vi "Main.vi"(11 "Module Admin":refnum<class "Delacor_lib_QMH_Module Admin.lvclass">) -> ()   [LabVIEW 2018, in "MB switches Module.lvlib"]
doc: "This template is based off of the Queued Message Handler design pattern and the Queued Message Handler project template that ships with LabVIEW.\n\nThe main difference is that the queue is private to this module and communication between modules is performed via Broadcast and Request events.\n\nRequest events are wrapped in public API methods and are handled in the Event Handling Loop (EHL) of this VI. Any module can register for Broadcast events sent by this module. The EHL generates messages based on user interface actions.\n\nThe Message Handling Loop (MHL) processes messages generated by the EHL, or by other messages. The messages are string values, so new messages can be added easily to the Message Cases case structure in the MHL. Each message cluster can also provide an optional value for Message Data, which is a variant that can be converted to whatever message-specific data is required.\n_____\nBased on DQMH Project Template 6.0.0.91."
uses:
  MB switches Module.lvlib
  <vilib>/Delacor/Delacor QMH/Libraries/Module Admin_class/Delacor_lib_QMH_Module Admin.lvclass
  Module Data--cluster.ctl
  <vilib>/NI/Modbus Library/API/Master/Modbus Master.lvclass
  Do Something Else and Wait for Reply Argument--cluster.ctl
  Do Something Else and Wait (Reply Payload)--cluster.ctl
  <vilib>/Delacor/Delacor QMH/Libraries/Message Queue_class/Delacor_lib_QMH_Message Queue.lvclass/Delacor_lib_QMH_Message Queue.ctl
  Stop Argument--cluster.ctl
  <vilib>/Delacor/Delacor QMH/Libraries/Module Admin_class/Delacor_lib_QMH_Module Admin.lvclass/Delacor_lib_QMH_Module Admin.ctl
  inst.Counter Argument--cluster.ctl
  inst.Counter (Reply Payload)--cluster.ctl
  inst.Optos Argument--cluster.ctl
  inst.Optos (Reply Payload)--cluster.ctl
  inst.mux10_1 Argument--cluster.ctl
  inst.mux6_1(3wires) Argument--cluster.ctl
  inst.Open Argument--cluster.ctl
  inst.Close Argument--cluster.ctl
  DMM I 0.5_10 Argument--cluster.ctl
  <vilib>/Utility/miscctls.llb/LVPointTypeDef.ctl
  Instrument Drivers/LV_driver_MBrelay/type defs/FGV enum.ctl
  <vilib>/Delacor/Delacor QMH/Libraries/Message Queue_class/Delacor_lib_QMH_Enqueue Message (Single).vi
  <vilib>/Delacor/Delacor QMH/Libraries/Module Admin_class/Delacor_lib_QMH_Get External Launch.vi
  <vilib>/Utility/error.llb/Error Cluster From Error Code.vi
  <vilib>/ErrorRing/Error Ring.xnode
  <vilib>/Delacor/Delacor QMH/Libraries/Message Queue_class/Delacor_lib_QMH_Message Queue.lvclass
  Instrument Drivers/LV_driver_MBrelay/MB Relay.lvlib
panel:
  in  "VISA resource name":refnum<visa-resource-name>="COM4"
  out "error out":errorcluster
  out "Status":string
  in  "Simulate MHL Error":bool
  in  "Simulate EHL Error":bool
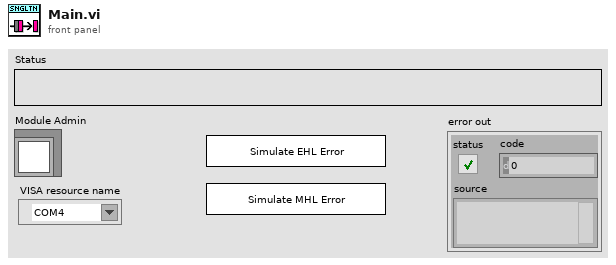
[diagram p1: front panel]
types:
  T1 = typedef "MB switches Module.lvlib/Request Events--cluster.ctl" = cluster{"Stop Module":refnum<user-event>, "Do Something Else and Wait for Reply":refnum<user-event>, "Show Panel":refnum<user-event>, "Hide Panel":refnum<user-event>, "Get Module Execution Status":refnum<user-event>, "Show Diagram":refnum<user-event>, "inst.Counter":refnum<user-event>, "inst.Open":refnum<user-event>, "inst.Close":refnum<user-event>, "inst.Optos":refnum<user-event>, "inst.mux10_1":refnum<user-event>, "inst.mux6_1(3wires)":refnum<user-event>, "DMM I 0.5_10":refnum<user-event>}
  T2 = typedef "MB switches Module.lvlib/Module Data--cluster.ctl" = cluster{"Status":string, "Modbus Master ref":refnum<class "Modbus Master.lvclass">}
  T3 = typedef "MB switches Module.lvlib/Do Something Else and Wait for Reply Argument--cluster.ctl" = cluster{"Do Something Else Msg":string, "X":dbl, "Wait Notifier":refnum<notifier>, "wait for reply":bool}
  T4 = enum32{"invalid lock state", "Not Locked", "Locked (No Password)", "Password-protected"}
  T5 = typedef "MB switches Module.lvlib/Stop Argument--cluster.ctl" = cluster{"Origin":string, "Exit via Stop Module Req?":bool, "Wait for Module to stop?":bool}
  T6 = typedef "MB switches Module.lvlib/inst.Counter Argument--cluster.ctl" = cluster{"Wait Notifier":refnum<notifier>, "wait for reply":bool}
  T7 = typedef "MB switches Module.lvlib/inst.Optos Argument--cluster.ctl" = cluster{"Wait Notifier":refnum<notifier>, "wait for reply":bool}
  T8 = typedef "MB switches Module.lvlib/inst.mux10_1 Argument--cluster.ctl" = cluster{"mux10_1(x6)_encode":enum16{"mux10_1_channel0", "mux10_1_channel1", "mux10_1_channel2", "mux10_1_channel3", "mux10_1_channel4", "mux10_1_channel5", "mux10_1_channel6", "mux10_1_channel7", "mux10_1_channel8", "mux10_1_channel9", "mux10_1_channel10"}}
  T9 = typedef "MB switches Module.lvlib/inst.mux6_1(3wires) Argument--cluster.ctl" = cluster{"mux6_1(3wires)_encode":enum16{"mux6-1_channel0", "mux6_1_channel1_0", "mux6_1_channel1_1", "mux6-1_channel1_2", "mux6_1_channel1_3", "mux6_1_channel2_0", "mux6_1_channel2_1", "mux6_1_channel2_2", "mux6_1_channel2_3", "mux6_1_channel3_0", "mux6_1_channel3_1", "mux6_1_channel3_2", "mux6_1_channel3_3", "mux6_1_channel4_0", "mux6_1_channel4_1", "mux6_1_channel4_2", "mux6_1_channel4_3", "mux6_1_channel5_0", "mux6_1_channel5_1", "mux6_1_channel5_2", "mux6_1_channel5_3", "mux6_1_channel6_0", "mux6_1_channel6_1", "mux6_1_channel6_2", "mux6_1_channel6_3"}}
  T10 = typedef "MB switches Module.lvlib/DMM I 0.5_10 Argument--cluster.ctl" = cluster{"mux2-1(DMM I) encode":enum16{"DMM I (0.5)", "DMM I (12)"}}
  T11 = typedef "LVPointTypeDef.ctl" = cluster{"Horizontal":i16, "Vertical":i16}
  T12 = enum32{"Invalid", "Standard", "Closed", "Hidden", "Minimized", "Maximized"}
  T13 = typedef "MB switches Module.lvlib/Do Something Else and Wait (Reply Payload)--cluster.ctl" = cluster{"Value":dbl, "error":errorcluster}
  T14 = typedef "MB switches Module.lvlib/inst.Counter (Reply Payload)--cluster.ctl" = cluster{"counter":u16, "inst.Counter_error":errorcluster}
  T15 = typedef "MB switches Module.lvlib/inst.Open Argument--cluster.ctl" = cluster{"VISA resource name":refnum<visa-resource-name>}
  T16 = typedef "MB Relay.lvlib/FGV enum.ctl" = enum16{"Write", "Read", "All OFF", "All ON"}
  T17 = typedef "MB switches Module.lvlib/inst.Close Argument--cluster.ctl" = cluster{"Boolean":bool}
  T18 = typedef "MB switches Module.lvlib/inst.Optos (Reply Payload)--cluster.ctl" = cluster{"Optos":bool[], "inst.Optos_error":errorcluster}
  T19 = enum16{"mux10_1_channel0", "mux10_1_channel1", "mux10_1_channel2", "mux10_1_channel3", "mux10_1_channel4", "mux10_1_channel5", "mux10_1_channel6", "mux10_1_channel7", "mux10_1_channel8", "mux10_1_channel9", "mux10_1_channel10"}
  T20 = enum16{"mux6-1_channel0", "mux6_1_channel1_0", "mux6_1_channel1_1", "mux6-1_channel1_2", "mux6_1_channel1_3", "mux6_1_channel2_0", "mux6_1_channel2_1", "mux6_1_channel2_2", "mux6_1_channel2_3", "mux6_1_channel3_0", "mux6_1_channel3_1", "mux6_1_channel3_2", "mux6_1_channel3_3", "mux6_1_channel4_0", "mux6_1_channel4_1", "mux6_1_channel4_2", "mux6_1_channel4_3", "mux6_1_channel5_0", "mux6_1_channel5_1", "mux6_1_channel5_2", "mux6_1_channel5_3", "mux6_1_channel6_0", "mux6_1_channel6_1", "mux6_1_channel6_2", "mux6_1_channel6_3"}
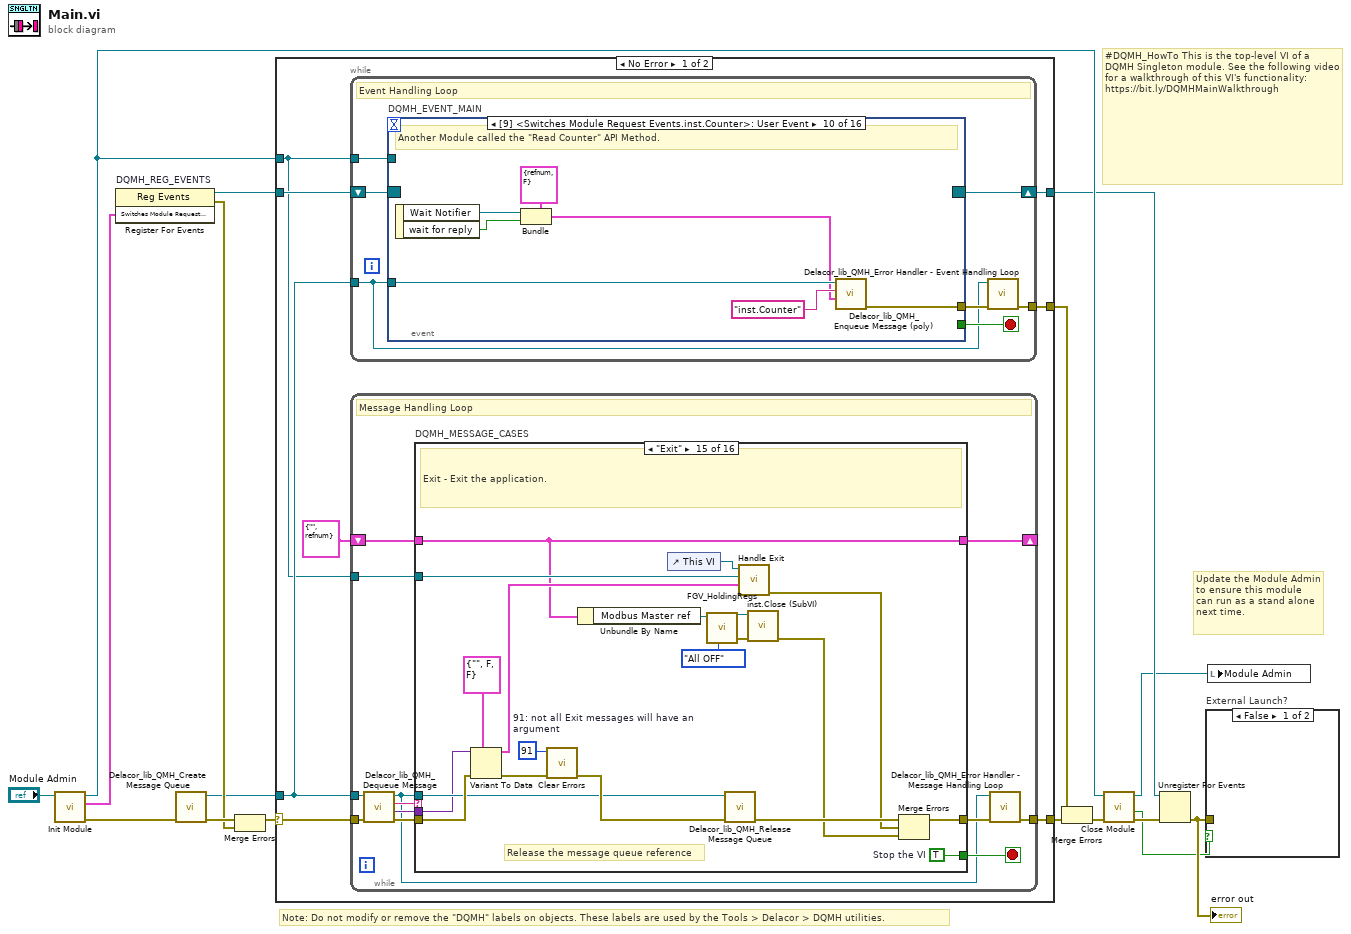
[diagram p0: block diagram]
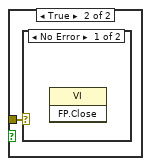
[diagram p2: hidden frame]
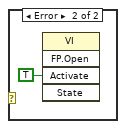
[diagram p3: hidden frame]
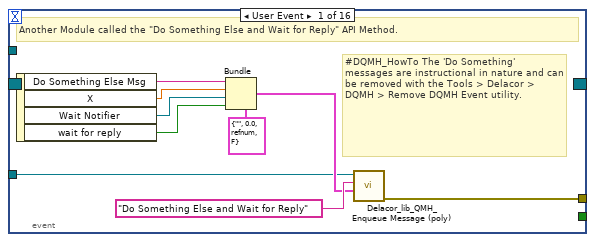
[diagram p4: hidden frame]
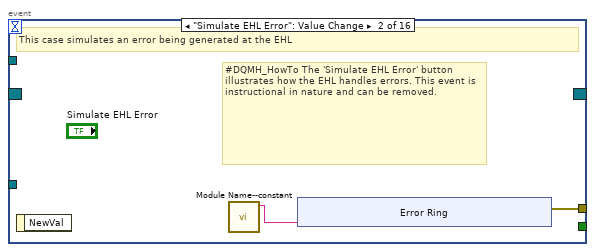
[diagram p5: hidden frame]
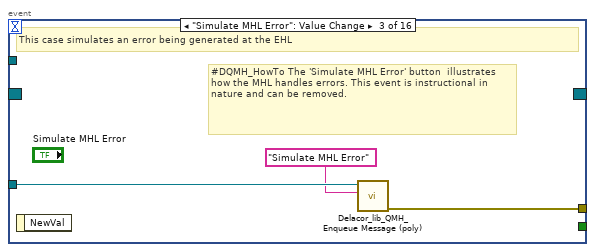
[diagram p6: hidden frame]
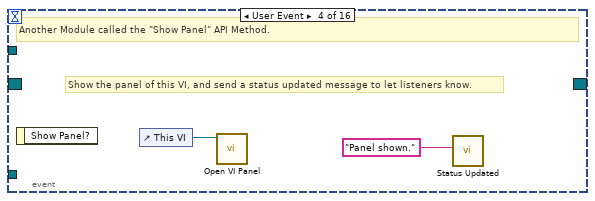
[diagram p7: hidden frame]
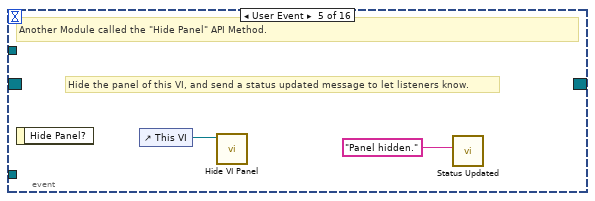
[diagram p8: hidden frame]
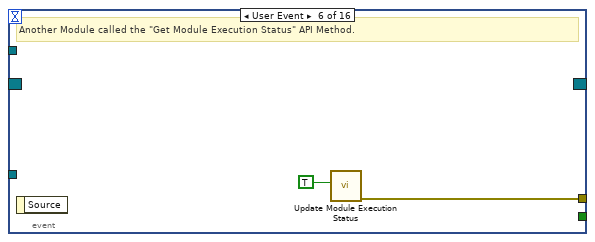
[diagram p9: hidden frame]
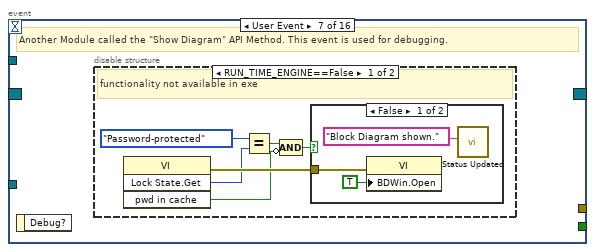
[diagram p10: hidden frame]
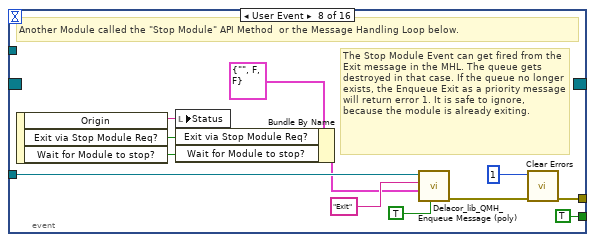
[diagram p13: hidden frame]
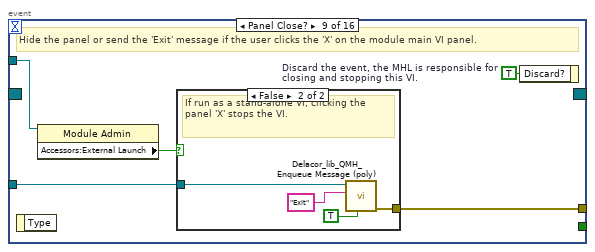
[diagram p14: hidden frame]
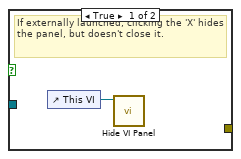
[diagram p15: hidden frame]
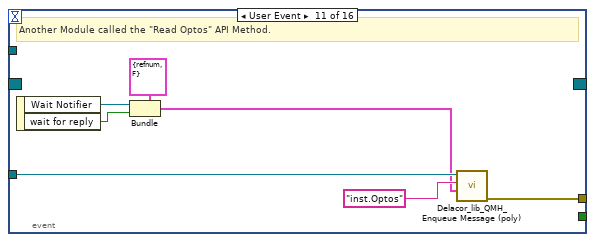
[diagram p16: hidden frame]
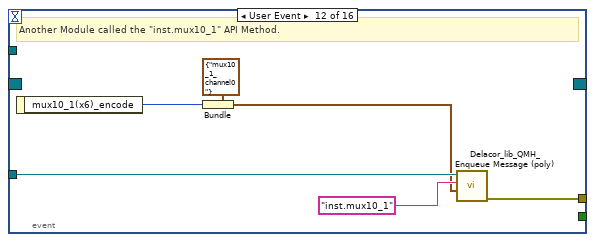
[diagram p17: hidden frame]
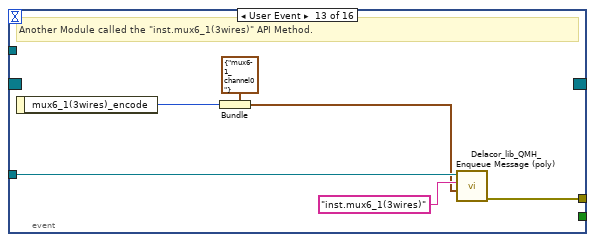
[diagram p18: hidden frame]
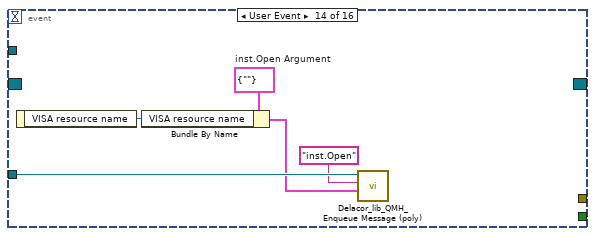
[diagram p19: hidden frame]
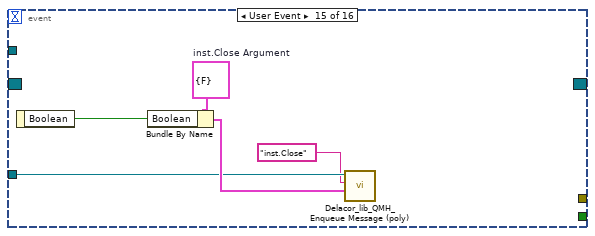
[diagram p20: hidden frame]
diagram:
  # "#DQMH_HowTo This is the top-level VI of a DQMH Singleton module. See the following video for a walkthrough of this VI's functionality: https://bit.ly/DQMHMainWalkthrough"
  # "Note: Do not modify or remove the \"DQMH\" labels on objects. These labels are used by the Tools > Delacor > DQMH utilities."
  # "Update the Module Admin to ensure this module can run as a stand alone next time."
  n1 = call "Init Module.vi"("Singleton Module Admin in"="Module Admin") -> ("error out"=w16:errorcluster, "Switches Module Request Events"=w2:T1, "Singleton Module Admin out"=w8:refnum<class "Delacor_lib_QMH_Module Admin.lvclass">)  [unwired: 8 in]
  n2 = register-events "DQMH_REG_EVENTS"(w2) -> (reference out=w1:refnum<event-registration>, error out=w9:errorcluster)  [unwired: 2 in]
  n3 = call <vilib>:"Delacor_lib_QMH_Create Message Queue.vi"("error in"=w16) -> ("error out"=w11:errorcluster, "Message Queue"=w6:refnum<class "Delacor_lib_QMH_Message Queue.lvclass">)  [unwired: 9 in]
  n4 = Merge Errors(w11, w9) -> (w10:errorcluster)
  n5 = case shown="No Error" w10 {
    selector: w10 -> [w23 w357]
    tunnel: [w25 w356] -> w17
    tunnel: [w22 w362] -> w7
    tunnel: w1 -> [w20 w362]
    tunnel: w6 -> [w19 w355]
    tunnel: [w24 _] -> w14
    tunnel: w8 -> [w18 w358]
    frame No Error {
      n6 = while {
        tunnel: w19 -> [w26]
        shift-right: [w29] -> w22
        shift-left: w20 -> [w30]
        tunnel: [w31] -> w24
        tunnel: w18 -> [w27]
        stop <- w28 stop-if-true
        # "Event Handling Loop"
        n7 = event "DQMH_EVENT_MAIN" shown="[9] <Switches Module Request Events.inst.Counter>: User Event" {
          selector: w30 -> [_ _ _ _ _ _ _ _ _ _ _ _ _ _ _ _]
          dyn-events: [_ _ _ _ _ _ _ _ _ _ _ _ _ _ _ _] -> w29
          timeout: _ -> [_ _ _ _ _ _ _ _ _ _ _ _ _ _ _ _]
          tunnel: [_ _ _ _ _ _ _ TRUE ("Discard?") _ _ _ _ _ _ _ _] -> w28
          tunnel: w26 -> [w34 _ w52 _ _ _ _ w76 w83 w97 w104 w110 w116 w121 w123 w132]
          tunnel: [w41 w43 w53 _ _ w59 _ w79 w85 w91 w98 w105 w111 _ _ w127] -> w32
          tunnel: w27 -> [_ _ _ _ _ _ _ _ w82 _ _ _ _ _ _ _]
          event User Event {
            # "#DQMH_HowTo The 'Do Something' messages are instructional in nature and can be removed with the Tools > Delacor > DQMH > Remove DQMH Event utility."
            # "Another Module called the \"Do Something Else and Wait for Reply\" API Method."
            n8 = event-data() -> ("Do Something Else Msg"=w37:string, "X"=w36:dbl, "Wait Notifier"=w35:refnum<notifier>, "wait for reply"=w33:bool)  [unwired: 1 in]
            n9 = Bundle(cluster=T3 {"Do Something Else Msg"="", "X"=0.0, "Wait Notifier"=refnum, "wait for reply"=FALSE} ("Do Something Else and Wait for Reply Argument"), "Do Something Else Msg"=w37, "X"=w36, "Wait Notifier"=w35, "wait for reply"=w33) -> (w38:T3)
            n10 = call-poly <vilib>:"Delacor_lib_QMH_Enqueue Message (poly).vi"("Message Data"=w38, "Message"="Do Something Else and Wait for Reply", "Message Queue in"=w34) -> ("error out"=w41:errorcluster)  [unwired: 7 in, 1 out]
          }
          event "Simulate EHL Error": Value Change {
            # "#DQMH_HowTo The 'Simulate EHL Error' button  illustrates how the EHL handles errors. This event is instructional in nature and can be removed."
            # "This case simulates an error being generated at the EHL"
            n11 = event-data() -> ()  [unwired: 1 in, 1 out]
            n12 = call "Module Name--constant.vi"() -> ("Module Name"=w42:string)  [unwired: 11 in]
            n13 = xnode "Error Ring"("parameter 0"=w42) -> ("error out"=w43:errorcluster)
          }
          event "Simulate MHL Error": Value Change {
            # "#DQMH_HowTo The 'Simulate MHL Error' button  illustrates how the MHL handles errors. This event is instructional in nature and can be removed."
            # "This case simulates an error being generated at the EHL"
            n14 = event-data() -> ()  [unwired: 1 in, 1 out]
            n15 = call-poly <vilib>:"Delacor_lib_QMH_Enqueue Message (poly).vi"("Message"="Simulate MHL Error", "Message Queue in"=w52) -> ("error out"=w53:errorcluster)  [unwired: 8 in, 1 out]
          }
          event User Event {
            # "Show the panel of this VI, and send a status updated message to let listeners know."
            # "Another Module called the \"Show Panel\" API Method."
            n16 = event-data() -> ()  [unwired: 1 in, 1 out]
            n17 = control-ref of="This VI"() -> (w55:refnum<vi>)
            n18 = call "Open VI Panel.vi"("VI"=w55) -> ()  [unwired: 10 in, 1 out]
            n19 = call "Status Updated.vi"("Status"="Panel shown." ("format string")) -> ()  [unwired: 10 in, 1 out]
          }
          event User Event {
            # "Hide the panel of this VI, and send a status updated message to let listeners know."
            # "Another Module called the \"Hide Panel\" API Method."
            n20 = event-data() -> ()  [unwired: 1 in, 1 out]
            n21 = control-ref of="This VI"() -> (w57:refnum<vi>)
            n22 = call "Hide VI Panel.vi"("VI"=w57) -> ()  [unwired: 10 in, 1 out]
            n23 = call "Status Updated.vi"("Status"="Panel hidden." ("format string")) -> ()  [unwired: 10 in, 1 out]
          }
          event User Event {
            # "Another Module called the \"Get Module Execution Status\" API Method."
            n24 = event-data() -> ()  [unwired: 1 in, 1 out]
            n25 = call "Update Module Execution Status.vi"("Running?"=TRUE) -> ("error out"=w59:errorcluster)  [unwired: 10 in]
          }
          event User Event {
            # "Another Module called the \"Show Diagram\" API Method. This event is used for debugging."
            n26 = event-data() -> ()  [unwired: 1 in, 1 out]
            n27 = disable-structure shown="RUN_TIME_ENGINE==False" {
              frame condition #0 (active) {
                # "functionality not available in exe"
                n28 = invoke class="VI" method="Lock State.Get"() -> (error out=w65:errorcluster, "Get Lock State"=w64:T4, "pwd in cache"=w61:bool)  [unwired: 4 in, 1 out]
                n29 = Equal?(x=T4."Password-protected", y=w64) -> (x = y?=w62:bool)
                n30 = Compound Arithmetic op=AND(w62, invert w61) -> (w60:bool)
                n31 = case shown="False" w60 {
                  tunnel: w65 -> [w68 _]
                  frame False {
                    n32 = property class="VI"(error in=w68, "BDWin.Open"=TRUE ("Block Diagram Window:Open")) -> ()  [unwired: 1 in, 2 out]
                    n33 = call "Status Updated.vi"("Status"="Block Diagram shown." ("format string")) -> ()  [unwired: 10 in, 1 out]
                  }
                  frame True {
                    # "Password-protected VI, and the password is not in the cache. Do not show the diagram."
                  }
                }
              }
              frame condition #1 {
              }
            }
          }
          event User Event {
            # "The Stop Module Event can get fired from the Exit message in the MHL. The queue gets destroyed in that case. If the queue no longer exists, the Enqueue Exit as a priority message will return error 1. It is safe to ignore, because the module is already exiting."
            # "Another Module called the \"Stop Module\" API Method  or the Message Handling Loop below."
            n34 = event-data() -> ("Origin"=w75:string, "Exit via Stop Module Req?"=w71:bool, "Wait for Module to stop?"=w70:bool)  [unwired: 1 in]
            n35 = local write "Status"(w75) -> ()
            n36 = Bundle By Name(cluster=T5 {"Origin"="", "Exit via Stop Module Req?"=FALSE, "Wait for Module to stop?"=FALSE} ("Stop Argument"), "Exit via Stop Module Req?"=w71, "Wait for Module to stop?"=w70) -> (w69:T5)
            n37 = call-poly <vilib>:"Delacor_lib_QMH_Enqueue Message (poly).vi"("Priority Message? (F)"=TRUE, "Message Data"=w69, "Message"="Exit", "Message Queue in"=w76) -> ("error out"=w80:errorcluster)  [unwired: 6 in, 1 out]
            n38 = call <vilib>:"Clear Errors.vi"("error in (no error)"=w80, "specific error code to clear (0: all)"=1) -> ("error out"=w79:errorcluster)  [unwired: 4 in, 1 out]
          }
          event Panel Close? {
            w84 = TRUE  # Discard the event, the MHL is responsible for closing and stopping this VI.
            # "Hide the panel or send the 'Exit' message if the user clicks the 'X' on the module main VI panel."
            n39 = event-data() -> ()  [unwired: 1 in, 1 out]
            n40 = property class="Module Admin"(reference=w82) -> ("Accessors:External Launch"=w81:bool)  [unwired: 1 in, 2 out]
            n41 = case shown="False" w81 {
              tunnel: w83 -> [_ w89]
              tunnel: [_ w90] -> w85
              frame True {
                # "If externally launched, clicking the 'X' hides the panel, but doesn't close it."
                n42 = control-ref of="This VI"() -> (w86:refnum<vi>)
                n43 = call "Hide VI Panel.vi"("VI"=w86) -> ()  [unwired: 10 in, 1 out]
              }
              frame False {
                # "If run as a stand-alone VI, clicking the panel 'X' stops the VI."
                n44 = call-poly <vilib>:"Delacor_lib_QMH_Enqueue Message (poly).vi"("Priority Message? (F)"=TRUE, "Message"="Exit", "Message Queue in"=w89) -> ("error out"=w90:errorcluster)  [unwired: 7 in, 1 out]
              }
            }
            n45 = event-data("Discard?"=w84) -> ()  [unwired: 1 in, 1 out]
          }
          event User Event {
            # "Another Module called the \"Read Counter\" API Method."
            n46 = event-data() -> ("Wait Notifier"=w93:refnum<notifier>, "wait for reply"=w92:bool)  [unwired: 1 in]
            n47 = Bundle(cluster=T6 {"Wait Notifier"=refnum, "wait for reply"=FALSE} ("Read Counter Argument"), "Wait Notifier"=w93, "wait for reply"=w92) -> (w94:T6)
            n48 = call-poly <vilib>:"Delacor_lib_QMH_Enqueue Message (poly).vi"("Message Data"=w94, "Message"="inst.Counter", "Message Queue in"=w97) -> ("error out"=w91:errorcluster)  [unwired: 7 in, 1 out]
          }
          event User Event {
            # "Another Module called the \"Read Optos\" API Method."
            n49 = event-data() -> ("Wait Notifier"=w100:refnum<notifier>, "wait for reply"=w99:bool)  [unwired: 1 in]
            n50 = Bundle(cluster=T7 {"Wait Notifier"=refnum, "wait for reply"=FALSE} ("Read Optos Argument"), "Wait Notifier"=w100, "wait for reply"=w99) -> (w101:T7)
            n51 = call-poly <vilib>:"Delacor_lib_QMH_Enqueue Message (poly).vi"("Message Data"=w101, "Message"="inst.Optos", "Message Queue in"=w104) -> ("error out"=w98:errorcluster)  [unwired: 7 in, 1 out]
          }
          event User Event {
            # "Another Module called the \"inst.mux10_1\" API Method."
            n52 = event-data() -> ("mux10_1(x6)_encode"=w106:T19)  [unwired: 1 in]
            n53 = Bundle(cluster=T8 {"mux10_1(x6)_encode"=enum."mux10_1_channel0"} ("inst.mux10_1 Argument"), "mux10_1(x6)_encode"=w106) -> (w107:T8)
            n54 = call-poly <vilib>:"Delacor_lib_QMH_Enqueue Message (poly).vi"("Message Data"=w107, "Message"="inst.mux10_1", "Message Queue in"=w110) -> ("error out"=w105:errorcluster)  [unwired: 7 in, 1 out]
          }
          event User Event {
            # "Another Module called the \"inst.mux6_1(3wires)\" API Method."
            n55 = event-data() -> ("mux6_1(3wires)_encode"=w112:T20)  [unwired: 1 in]
            n56 = Bundle(cluster=T9 {"mux6_1(3wires)_encode"=enum."mux6-1_channel0"} ("inst.mux6_1(3wires) Argument"), "mux6_1(3wires)_encode"=w112) -> (w113:T9)
            n57 = call-poly <vilib>:"Delacor_lib_QMH_Enqueue Message (poly).vi"("Message Data"=w113, "Message"="inst.mux6_1(3wires)", "Message Queue in"=w116) -> ("error out"=w111:errorcluster)  [unwired: 7 in, 1 out]
          }
          event User Event {
            w119 = T15 {"VISA resource name"=""}  # inst.Open Argument
            n58 = event-data() -> ("VISA resource name"=w118:refnum<visa-resource-name>)  [unwired: 1 in]
            n59 = Bundle By Name(cluster=w119, "VISA resource name"=w118) -> (w117:T15)
            n60 = call-poly <vilib>:"Delacor_lib_QMH_Enqueue Message (poly).vi"("Message Data"=w117, "Message"="inst.Open", "Message Queue in"=w121) -> ()  [unwired: 7 in, 2 out]
          }
          event User Event {
            w126 = T17 {"Boolean"=FALSE}  # inst.Close Argument
            n61 = event-data() -> ("Boolean"=w125:bool)  [unwired: 1 in]
            n62 = Bundle By Name(cluster=w126, "Boolean"=w125) -> (w124:T17)
            n63 = call-poly <vilib>:"Delacor_lib_QMH_Enqueue Message (poly).vi"("Message Data"=w124, "Message"="inst.Close", "Message Queue in"=w123) -> ()  [unwired: 7 in, 2 out]
          }
          event User Event {
            # "Another Module called the \"DMM I 0.5_10\" API Method."
            n64 = event-data() -> ("mux2-1(DMM I) encode"=w128:enum16{"DMM I (0.5)", "DMM I (12)"})  [unwired: 1 in]
            n65 = Bundle(cluster=T10 {"mux2-1(DMM I) encode"=enum."DMM I (0.5)"} ("DMM I 0.5_10 Argument"), "mux2-1(DMM I) encode"=w128) -> (w129:T10)
            n66 = call-poly <vilib>:"Delacor_lib_QMH_Enqueue Message (poly).vi"("Message Data"=w129, "Message"="DMM I 0.5_10", "Message Queue in"=w132) -> ("error out"=w127:errorcluster)  [unwired: 7 in, 1 out]
          }
        }
        n67 = call-dynamic "Delacor_lib_QMH_Error Handler - Event Handling Loop.vi"("error in"=w32, "Message Queue in"=w26) -> ("dup error in"=w31:errorcluster)  [unwired: 8 in, 1 out]
      }
      n68 = while {
        tunnel: w19 -> [w135]
        shift-right: [w139] -> _
        shift-left: T2 {"Status"="", "Modbus Master ref"=refnum} ("Data Cluster") -> [w140]
        tunnel: w23 -> [w143]
        tunnel: [w141] -> w25
        tunnel: w18 -> [w133]
        stop <- w138 stop-if-true
        # "Message Handling Loop"
        n69 = call-dynamic "Delacor_lib_QMH_Dequeue Message.vi"("error in"=w143, "Message Queue in"=w135) -> ("error out"=w142:errorcluster, "Message Data"=w136:variant, "Message"=w137:string, "Message Queue out"=w134:refnum<class "Delacor_lib_QMH_Message Queue.lvclass">)  [unwired: 6 in]
        n70 = case "DQMH_MESSAGE_CASES" shown="\"Exit\"" w137 {
          selector: w137 -> [_ _ _ _ _ _ _ _ _ _ _ _ _ _ _ w342]
          tunnel: w134 -> [_ _ _ _ _ _ _ _ _ _ _ _ _ w307 w334 _]
          tunnel: w142 -> [w168 w172 w191 w217 w230 w241 w255 w267 w277 w287 w290 w292 w297 w314 w340 w344]
          tunnel: [w167 w172 w190 w209 w221 w231 w247 w258 w269 w279 w289 w292 w296 w310 w337 w345] -> w144
          tunnel: w140 -> [w147 w171 w188 w208 w223 w236 w246 w262 w273 w283 w288 w291 w294 w309 w322 w343]
          tunnel: [w158 w171 w188 w208 w224 w236 w246 w262 w273 w283 w288 w291 w294 w309 w322 w343] -> w139
          tunnel: [_ _ _ _ _ _ _ _ _ _ _ _ _ _ w333 _] -> w138
          tunnel: w136 -> [_ _ w185 w216 w229 w240 w254 w266 w276 w286 _ _ _ w308 w332 _]
          tunnel: w133 -> [w159 _ _ _ _ _ _ _ _ _ _ _ _ w306 w327 _]
          frame "Initialize" {
            w154 = "Initial Message" ("Initial Message")
            # "Initialize - Any operation that needs to be done before the module can receive messages. Synchronize Caller Events.vi will inform Start Module.vi that the module has launched and is ready to receive messages. Module Did Init.vi will broadcast that the module initialized."
            n71 = call "Synchronize Caller Events.vi"("error in (no error)"=w168, "Singleton Module Admin in"=w159) -> ("error out"=w152:errorcluster, "Singleton Module Admin out"=w155:refnum<class "Delacor_lib_QMH_Module Admin.lvclass">)  [unwired: 8 in]
            n72 = property class="Module Admin"(reference=w155) -> ("Accessors:External Launch"=w163:bool)  [unwired: 1 in, 2 out]
            n73 = call "inst.Open.vi"("unit ID in"=u8 1, "VISA resource name"="VISA resource name") -> ("error out"=w145:errorcluster, "Modbus Master out"=w146:refnum<class "Modbus Master.lvclass">)  [unwired: 8 in]
            n74 = Bundle By Name(cluster=w147, "Modbus Master ref"=w146) -> (w148:T2)
            n75 = Select(t=T12."Hidden" ("State"), s=w163, f=T12."Standard" ("State")) -> (s? t:f=w160:T12)
            n76 = Merge Errors(w152, w145) -> (w151:errorcluster)
            n77 = call "Module Name--constant.vi"() -> ("Module Name"=w166:string)  [unwired: 11 in]
            n78 = property class="VI"("Front Panel.Title"=w166) -> (reference out=w165:refnum<vi>, error out=w170:errorcluster)  [unwired: 2 in]
            n79 = call "Module Name--constant.vi"() -> ("Module Name"=w156:string)  [unwired: 11 in]
            n80 = invoke class="VI" method="FP.Open"(reference=w165, error in=w170, "State"=w160) -> (reference out=w164:refnum<vi>, error out=w169:errorcluster)  [unwired: 2 in, 3 out]
            n81 = Bundle By Name(cluster=w148, "Status"=w154) -> (w158:T2)
            n82 = call "Module Did Init.vi"("error in (no error)"=w151, "Initialized?"=TRUE, "Origin"=w156) -> ("error out"=w167:errorcluster)  [unwired: 8 in]
            n83 = invoke class="VI" method="FP.Center"(reference=w164, error in=w169) -> ()  [unwired: 1 in, 3 out]
            n84 = property on="Pane" class="Pane"("Origin"=T11 {"Horizontal"=0, "Vertical"=0}) -> ()  [unwired: 2 in, 2 out]
            "Status" <- w154
          }
          frame "---Module Specific---" {
            # "Separator -- The following cases handle messages specific to this Module."
          }
          frame "Do Something Else and Wait for Reply" {
            w180 = "X(%.2f)+Offset(%.2f)=%.2f"  # status message format string
            # "#DQMH_HowTo The 'Do Something' messages are instructional in nature and can be removed."
            # "Send back X with a random offset"
            # "Do Something Else and Wait for Reply - Replace this message with functionality for your own application. Note that this message must fire a notifier to let callers know it has finished execution, and it returns an error if the 'Value' is negative."
            n85 = Random Number (0-1)() -> (number: 0 to 1=w182:dbl)
            n86 = Variant To Data(error in=w191, type=T3 {"Do Something Else Msg"="", "X"=0.0, "Wait Notifier"=refnum, "wait for reply"=FALSE} ("Do Something Else and Wait for Reply Argument"), Variant=w185) -> (data=w186:T3, error out=w189:errorcluster)
            n87 = Unbundle By Name(w186) -> ("Wait Notifier"=w173:refnum<notifier>, "Do Something Else Msg"=w184:string, "X"=w181:dbl, "wait for reply"=w177:bool)
            n88 = Add(x=w182, y=w181) -> (x+y=w176:dbl)
            n89 = Less Than 0?(x=w176) -> (x < 0?=w179:bool)
            n90 = Format Into String(format string=w180, initial string=w184, w181, w182, w176) -> (resulting string=w178:string)  [unwired: 1 in, 1 out]
            n91 = case shown="True" w179 {
              tunnel: [_ w198] -> w174
              frame False {
              }
              frame True {
                n92 = xnode "Error Ring"() -> ("error out"=w198:errorcluster)
              }
            }
            n93 = Bundle By Name(cluster=T13 {"Value"=0.0, "error"={"status"=FALSE, "code"=0, "source"=""}} ("notification"), "error"=w174, "Value"=w176) -> (w175:T13)
            n94 = local write "Status"(w178) -> ()
            n95 = call "Status Updated.vi"("Status"=w178) -> ()  [unwired: 10 in, 1 out]
            n96 = case shown="True" w177 {
              tunnel: w175 -> [_ w194]
              tunnel: w173 -> [_ w193]
              frame False {
              }
              frame True {
                # "Simulate an operation that requires a wait."
                n97 = flat-sequence {
                  tunnel: w194 -> [w197]
                  tunnel: w193 -> [w196]
                  tunnel: w192 -> [_]
                  frame #0 {
                    n98 = Send Notification(notification=w197, notifier=w196) -> ()  [unwired: 1 in, 2 out]
                  }
                }
                n99 = Wait (ms)(milliseconds to wait=u32 1000) -> (millisecond timer value=w192:u32)
              }
            }
            n100 = Merge Errors(w189, w174) -> (w190:errorcluster)
          }
          frame "inst.Counter" {
            # "Read Internal Counter to check state of MCU"
            n101 = Variant To Data(error in=w217, type=T6 {"Wait Notifier"=refnum, "wait for reply"=FALSE} ("Read Counter Argument"), Variant=w216) -> (data=w214:T6, error out=w205:errorcluster)
            n102 = Unbundle By Name(w208) -> ("Modbus Master ref"=w207:refnum<class "Modbus Master.lvclass">)
            n103 = Unbundle By Name(w214) -> ("Wait Notifier"=w213:refnum<notifier>, "wait for reply"=w212:bool)
            n104 = call "inst.counter.vi"("Modbus master in"=w207) -> ("error out"=w204:errorcluster, "counter"=w206:u16)  [unwired: 8 in, 1 out]
            n105 = Bundle By Name(cluster=T14 {"counter"=0, "inst.Counter_error"={"status"=FALSE, "code"=0, "source"=""}} ("Read Counter (Reply Payload)"), "counter"=w206) -> (w211:T14)
            n106 = case shown="True" w212 {
              tunnel: w213 -> [_ w219]
              tunnel: w211 -> [_ w218]
              frame False {
              }
              frame True {
                n107 = Send Notification(notification=w218, notifier=w219) -> ()  [unwired: 1 in, 2 out]
              }
            }
            n108 = Merge Errors(w205, w204) -> (w209:errorcluster)
          }
          frame "inst.Open" {
            # "send COMport name to Module and Open Modbus Insstance"
            n109 = Variant To Data(error in=w230, type=T15 {"VISA resource name"=""} ("Open COM Argument"), Variant=w229) -> (data=w227:T15, error out=w220:errorcluster)
            n110 = Unbundle By Name(w227) -> ("VISA resource name"=w226:refnum<visa-resource-name>)
            n111 = call "inst.Open.vi"("VISA resource name"=w226) -> ("error out"=w222:errorcluster, "Modbus Master out"=w225:refnum<class "Modbus Master.lvclass">)  [unwired: 9 in]
            n112 = Bundle By Name(cluster=w223, "Modbus Master ref"=w225) -> (w224:T2)
            n113 = Merge Errors(w220, w222) -> (w221:errorcluster)
          }
          frame "inst.Close" {
            # "Shut down all Relays and Close COM port"
            n114 = Variant To Data(error in=w241, type=T17 {"Boolean"=FALSE} ("Close COM Argument"), Variant=w240) -> (error out=w233:errorcluster)  [unwired: 1 out]
            n115 = Unbundle By Name(w236) -> ("Modbus Master ref"=w238:refnum<class "Modbus Master.lvclass">)
            n116 = call "FGV_HoldingRegs.vi"("FGV_enum"=FGV_enum."All OFF", "Modbus master in"=w238) -> ("error out"=w235:errorcluster, "Modbus master out"=w234:refnum<class "Modbus Master.lvclass">)  [unwired: 7 in, 1 out]
            n117 = call "inst.Close (SubVI).vi"("error in (no error)"=w235, "Modbus Master in"=w234) -> ("error out"=w232:errorcluster)  [unwired: 9 in]
            n118 = Merge Errors(w233, w232) -> (w231:errorcluster)
          }
          frame "inst.Optos" {
            # "Read 64 optos DIs"
            n119 = Variant To Data(error in=w255, type=T7 {"Wait Notifier"=refnum, "wait for reply"=FALSE} ("Read Optos Argument"), Variant=w254) -> (data=w252:T7, error out=w244:errorcluster)
            n120 = Unbundle By Name(w246) -> ("Modbus Master ref"=w245:refnum<class "Modbus Master.lvclass">)
            n121 = Unbundle By Name(w252) -> ("Wait Notifier"=w251:refnum<notifier>, "wait for reply"=w250:bool)
            n122 = call "inst.Optos.vi"("error in (no error)"=w244, "Modbus master in"=w245) -> ("error out"=w243:errorcluster, "optos"=w242:bool[])  [unwired: 7 in, 1 out]
            n123 = Bundle By Name(cluster=T18 {"Optos"=[], "inst.Optos_error"={"status"=FALSE, "code"=0, "source"=""}} ("Read Optos (Reply Payload)"), "Optos"=w242, "inst.Optos_error"=w243) -> (w249:T18)
            n124 = Merge Errors(w244, w243) -> (w247:errorcluster)
            n125 = case shown="True" w250 {
              tunnel: w251 -> [_ w257]
              tunnel: w249 -> [_ w256]
              frame False {
              }
              frame True {
                n126 = Send Notification(notification=w256, notifier=w257) -> ()  [unwired: 1 in, 2 out]
              }
            }
          }
          frame "inst.mux10_1" {
            # "Connect DRV output to LED loads"
            n127 = Variant To Data(error in=w267, type=T8 {"mux10_1(x6)_encode"=enum."mux10_1_channel0"} ("inst.mux10_1 Argument"), Variant=w266) -> (data=w264:T8, error out=w259:errorcluster)
            n128 = Unbundle By Name(w264) -> ("mux10_1(x6)_encode"=w263:T19)
            n129 = Unbundle By Name(w262) -> ("Modbus Master ref"=w261:refnum<class "Modbus Master.lvclass">)
            n130 = call "inst.mux10.1(x6).vi"("mux10_1(x6)_encode"=w263, "Modbus Master in"=w261) -> ("error out"=w260:errorcluster)  [unwired: 8 in, 1 out]
            n131 = Merge Errors(w259, w260) -> (w258:errorcluster)
          }
          frame "inst.mux6_1(3wires)" {
            # "connect Led DRV to DMM inputs"
            n132 = Variant To Data(error in=w277, type=T9 {"mux6_1(3wires)_encode"=enum."mux6-1_channel0"} ("inst.mux6_1(3wires) Argument"), Variant=w276) -> (data=w274:T9, error out=w270:errorcluster)
            n133 = Unbundle By Name(w273) -> ("Modbus Master ref"=w272:refnum<class "Modbus Master.lvclass">)
            n134 = Unbundle By Name(w274) -> ("mux6_1(3wires)_encode"=w271:T20)
            n135 = call "inst.mux6.1(3wires).vi"("mux6_1(3wires)_encode"=w271, "Modbus Master in"=w272) -> ("error out"=w268:errorcluster)  [unwired: 8 in, 1 out]
            n136 = Merge Errors(w270, w268) -> (w269:errorcluster)
          }
          frame "DMM I 0.5_10" {
            # "DMM config Current fuse 0.5 or 10A"
            n137 = Variant To Data(error in=w287, type=T10 {"mux2-1(DMM I) encode"=enum."DMM I (0.5)"} ("DMM I 0.5_10 Argument"), Variant=w286) -> (data=w284:T10, error out=w281:errorcluster)
            n138 = Unbundle By Name(w284) -> ("mux2-1(DMM I) encode"=w278:enum16{"DMM I (0.5)", "DMM I (12)"})
            n139 = Unbundle By Name(w283) -> ("Modbus Master ref"=w282:refnum<class "Modbus Master.lvclass">)
            n140 = call "inst.DMM (Current INPUT).vi"("mux2-1(DMM I) encode"=w278, "Modbus Master in"=w282) -> ("error out"=w280:errorcluster)  [unwired: 8 in, 1 out]
            n141 = Merge Errors(w281, w280) -> (w279:errorcluster)
          }
          frame "---Copy This Frame---" {
            # "Duplicate this frame when creating new messages.  Change this comment in the duplicated frame to describe this message."
            n142 = Merge Errors(w290) -> (w289:errorcluster)
          }
          frame "---Exit and Error Handling---" {
            # "Separator - The following cases handle errors and exit messages."
          }
          frame "Simulate MHL Error" {
            # "#DQMH_HowTo The 'Simulate MHL Error' button  illustrates how the MHL handles errors. This event is instructional in nature and can be removed."
            # "Simulate an error occurring at the MHL"
            n143 = call "Module Name--constant.vi"() -> ("Module Name"=w293:string)  [unwired: 11 in]
            n144 = xnode "Error Ring"("parameter 0"=w293) -> ("error out"=w295:errorcluster)
            n145 = Merge Errors(w297, w295) -> (w296:errorcluster)
          }
          frame "Error" {
            # "#CodeRecommended - If you ever change the name of this \"Error\" message, you'll need to update the name in the Check Loop Error.vi as well."
            # "#CodeRecommended - If the module is running in standalone mode (External Launch = FALSE), this code will pop up an error dialog and call the 'Exit' message if an error occurs. Add more fine-grained error handling here."
            # "Error - Check the error message data and respond accordingly. This message is sent by the \"Error Handler\" VIs at the end of each loop in this application."
            n146 = property class="Module Admin"(reference=w306) -> ("Accessors:External Launch"=w305:bool)  [unwired: 1 in, 2 out]
            n147 = Variant To Data(error in=w314, type=errorcluster {"status"=FALSE, "code"=0, "source"=""} ("error constant"), Variant=w308) -> (data=w315:errorcluster, error out=w312:errorcluster)
            n148 = call "Error Reported.vi"("Error"=w315) -> ()  [unwired: 10 in, 1 out]
            n149 = case shown="False" w305 {
              tunnel: [w320 _] -> w311
              tunnel: w307 -> [w318 _]
              tunnel: w315 -> [w319 _]
              frame False {
                # "If the module is running standalone, then pop up an error dialog and call the \"Exit\" message."
                n150 = call <vilib>:"Simple Error Handler.vi"("error in (no error)"=w319) -> ()  [unwired: 4 in, 5 out]
                n151 = call-poly <vilib>:"Delacor_lib_QMH_Enqueue Message (poly).vi"("Priority Message? (F)"=TRUE, "Message"="Exit", "Message Queue in"=w318) -> ("error out"=w320:errorcluster)  [unwired: 7 in, 1 out]
              }
              frame True {
                # "If the module was launched externally, calling the Error Reported broadcast VI is the only action performed by the \"Error\" message. The module's caller can then process the error appropriately."
              }
            }
            n152 = Merge Errors(w312, w311) -> (w310:errorcluster)
            n153 = local write "error out"(w310) -> ()
          }
          frame "Exit" {
            w331 = 91  # 91: not all Exit messages will have an argument
            w333 = TRUE  # Stop the VI
            # "Release the message queue reference"
            # "Exit - Exit the application."
            n154 = Variant To Data(error in=w340, type=T5 {"Origin"="", "Exit via Stop Module Req?"=FALSE, "Wait for Module to stop?"=FALSE} ("Stop Argument"), Variant=w332) -> (data=w329:T5, error out=w336:errorcluster)
            n155 = call <vilib>:"Clear Errors.vi"("error in (no error)"=w336, "specific error code to clear (0: all)"=w331) -> ("error out"=w339:errorcluster)  [unwired: 4 in, 1 out]
            n156 = Unbundle By Name(w322) -> ("Modbus Master ref"=w326:refnum<class "Modbus Master.lvclass">)
            n157 = control-ref of="This VI"() -> (w328:refnum<vi>)
            n158 = call "FGV_HoldingRegs.vi"("FGV_enum"=FGV_enum."All OFF", "Modbus master in"=w326) -> ("error out"=w325:errorcluster, "Modbus master out"=w324:refnum<class "Modbus Master.lvclass">)  [unwired: 7 in, 1 out]
            n159 = call-dynamic "Delacor_lib_QMH_Release Message Queue.vi"("error in"=w339, "Message Queue"=w334) -> ("error out"=w338:errorcluster)  [unwired: 9 in]
            n160 = call "Handle Exit.vi"("Stop Argument"=w329, "Admin in"=w327, "VI reference"=w328) -> ("error out"=w335:errorcluster)  [unwired: 7 in, 1 out]
            n161 = call "inst.Close (SubVI).vi"("error in (no error)"=w325, "Modbus Master in"=w324) -> ("error out"=w321:errorcluster)  [unwired: 9 in]
            n162 = Merge Errors(w338, w335, w321) -> (w337:errorcluster)
          }
          frame Default {
            # "'Default' case only runs if there is a message that isn't defined in any of the other cases.  Output a programming error."
            n163 = call "Module Name--constant.vi"() -> ("Module Name"=w341:string)  [unwired: 11 in]
            n164 = xnode "Error Ring"("parameter 0"=w342, "parameter 1"=w341) -> ("error out"=w346:errorcluster)
            n165 = Merge Errors(w344, w346) -> (w345:errorcluster)
          }
        }
        n166 = call-dynamic "Delacor_lib_QMH_Error Handler - Message Handling Loop.vi"("error in"=w144, "Message Queue in"=w134) -> ("dup error in"=w141:errorcluster)  [unwired: 8 in, 1 out]
      }
    }
    frame Error {
      # "Synchronize Caller Events.vi will inform Start Module.vi that the module has launched and will let the code calling Start Module.vi register for broadcasts and would permit the caller receive the broadcast that an error occurred at launch time."
      n167 = call-dynamic "Delacor_lib_QMH_Release Message Queue.vi"("error in"=w357, "Message Queue"=w355) -> ("error out"=w356:errorcluster)  [unwired: 9 in]
      n168 = call "Synchronize Caller Events.vi"("Singleton Module Admin in"=w358) -> ("error out"=w363:errorcluster)  [unwired: 9 in, 1 out]
      n169 = call "Module Name--constant.vi"() -> ("Module Name"=w361:string)  [unwired: 11 in]
      n170 = Format Into String(format string="An error occurred during initialization. %s is no longer running.", w361) -> (resulting string=w359:string)  [unwired: 2 in, 1 out]
      n171 = Merge Errors(w356, w363) -> (w364:errorcluster)
      n172 = call "Error Reported.vi"("Additional Information"=w359, "Error"=w364) -> ()  [unwired: 9 in, 1 out]
    }
  }
  n173 = Merge Errors(w14, w17) -> (w13:errorcluster)
  n174 = call "Close Module.vi"("error in (no error)"=w13, "Module Admin in"=w8) -> ("error out"=w15:errorcluster, "External Launch"=w3:bool, "Module Admin out"=w4:refnum<class "Delacor_lib_QMH_Module Admin.lvclass">)  [unwired: 7 in]
  n175 = Unregister For Events(event registration refnum=w7, error in=w15) -> (error out=w12:errorcluster)
  "error out" <- w12
  n176 = case "External Launch?" shown="False" w3 {
    tunnel: w12 -> [_ w365]
    frame False {
    }
    frame True {
      n177 = case shown="No Error" w365 {
        frame No Error {
          n178 = invoke class="VI" method="FP.Close"() -> ()  [unwired: 3 in, 3 out]
        }
        frame Error {
          n179 = invoke class="VI" method="FP.Open"("Activate"=TRUE ("Activate?")) -> ()  [unwired: 4 in, 5 out]
        }
      }
    }
  }
  n180 = local write "Module Admin"(w4) -> ()
